vi "resonant.display queue to fp display_MD.vi"() -> ()   [LabVIEW 2012]
uses:
  <vilib>/Utility/VariantDataType/Type.ctl
  GFG/GFGnumericGet.vi
  GFG/GFGbooleanGet.vi
  GFG/GFGImageRefsGet.vi
  GFG/GFGDisplayRefsGet.vi
  GFG/GFG library.lvlib
  <vilib>/Utility/VariantDataType/VariantType.lvlib
panel:
  out "error out 3":errorcluster
  out "error out 2":errorcluster
  out "size(s)":i32[](array[numeric])
  out "# elements in display data queue":i32
  out "error out":errorcluster
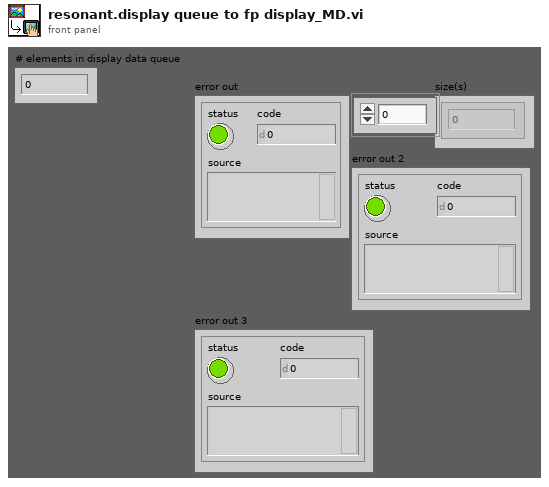
[diagram p1: front panel]
types:
  T1 = cluster{"NewVal":bool, "Event Registration Refnum":refnum<event-registration>}
  T2 = cluster{"Channel 1 small":refnum<vi>, "Channel 2 small":refnum<vi>, "Channel 3 small":refnum<vi>, "Channel 4 small":refnum<vi>, "Channel 1 large":refnum<vi>, "Channel 2 large":refnum<vi>, "Channel 3 large":refnum<vi>, "Channel 4 large":refnum<vi>, "RGB overlay":refnum<vi>, "ROI Image display":refnum<vi>, "arb line scan display":refnum<vi>, "Channel 5 large":refnum<vi>}
  T3 = typedef "IMAQ Image.ctl" = refnum<image>
  T4 = cluster{"Channel 1 small":T3, "Channel 2 small":T3, "Channel 3 small":T3, "Channel 4 small":T3, "Channel 1 large":T3, "Channel 2 large":T3, "Channel 3 large":T3, "Channel 4 large":T3, "RGB overlay":T3, "ROI Image display":T3, "arb line scan display":T3, "Channel 5 large":T3}
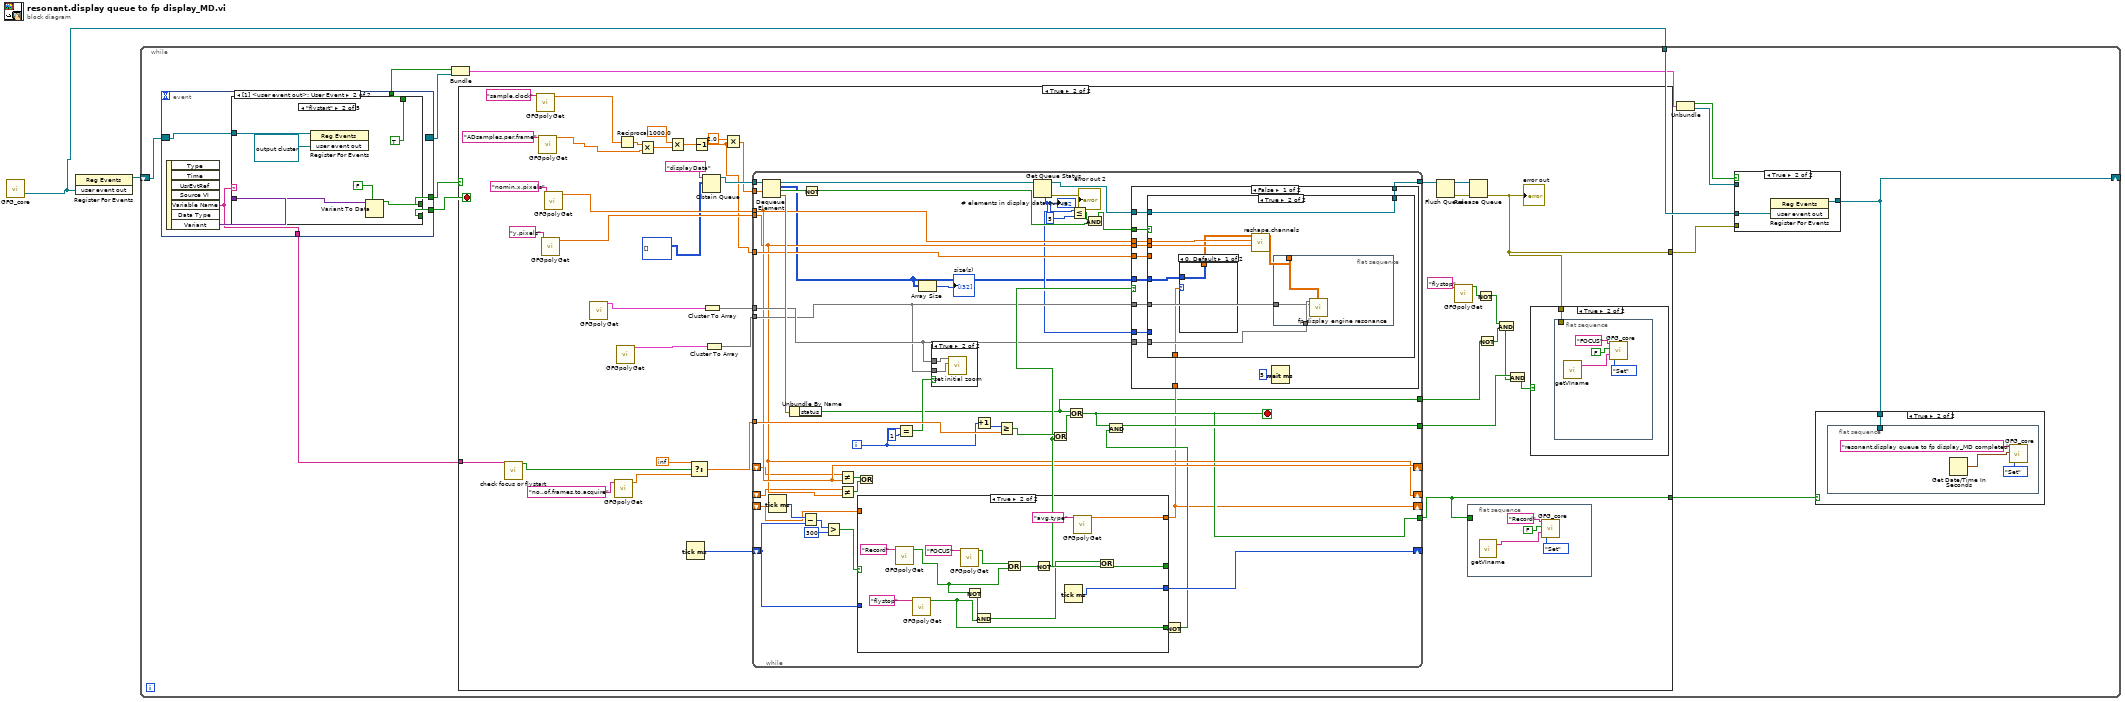
[diagram p0: block diagram]
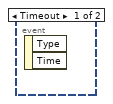
[diagram p4: hidden frame]
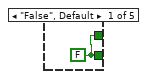
[diagram p5: hidden frame]
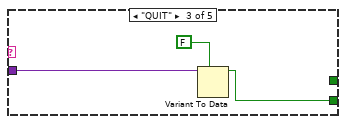
[diagram p6: hidden frame]
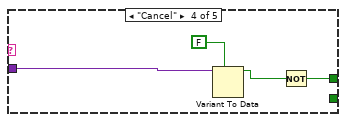
[diagram p7: hidden frame]
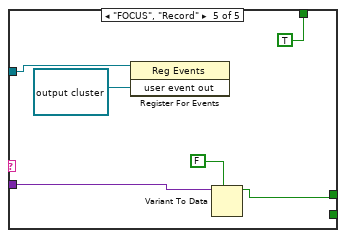
[diagram p8: hidden frame]
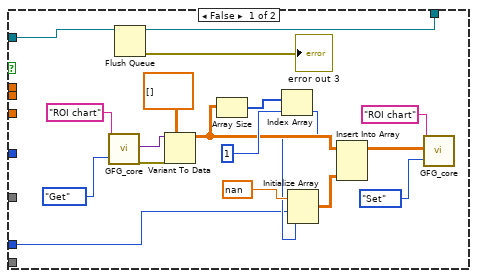
[diagram p12: hidden frame]
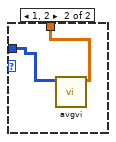
[diagram p13: hidden frame]
diagram:
  n1 = call "GFG_core.vi"() -> ("user event out"=w2:refnum<user-event>)  [unwired: 13 in, 6 out]
  n2 = register-events(w2) -> (reference out=w1:refnum<event-registration>)  [unwired: 2 in, 1 out]
  n3 = while {
    shift-right: [w3] -> _
    shift-left: w1 -> [w11]
    tunnel: w2 -> [w13]
    stop <- w14 stop-if-true
    n4 = event shown="[1] <user event out>: User Event" {
      selector: w11 -> [_ w24]
      dyn-events: [_ _] -> w9
      timeout: _ -> [_ _]
      tunnel: [_ w28] -> w15
      tunnel: [_ w27] -> w14
      tunnel: [_ w25] -> w5
      tunnel: [_ w23] -> w10
      event Timeout {
        n5 = event-data() -> ()  [unwired: 1 in, 2 out]
      }
      event User Event {
        n6 = event-data() -> ("Variable Name"=w25:string, "Variant"=w26:variant)  [unwired: 1 in, 5 out]
        n7 = case shown="\"flystart\"" w25 {
          tunnel: [w29 w33 _ w39 w46] -> w28
          tunnel: [w29 _ w36 _ _] -> w27
          tunnel: w26 -> [_ w34 w38 w41 w47]
          tunnel: w24 -> [_ w31 _ _ w44]
          tunnel: [_ TRUE ("NewVal") _ _ TRUE ("NewVal")] -> w23
          frame "False", Default {
            w29 = FALSE ("NewVal")
          }
          frame "flystart" {
            n8 = register-events(reference=w31, refnum<user-event> refnum ("user event out")) -> ()  [unwired: 1 in, 2 out]
            n9 = Variant To Data(type=FALSE ("NewVal"), Variant=w34) -> (data=w33:bool)  [unwired: 1 in, 1 out]
          }
          frame "QUIT" {
            n10 = Variant To Data(type=FALSE ("NewVal"), Variant=w38) -> (data=w36:bool)  [unwired: 1 in, 1 out]
          }
          frame "Cancel" {
            n11 = Variant To Data(type=FALSE ("NewVal"), Variant=w41) -> (data=w40:bool)  [unwired: 1 in, 1 out]
            n12 = Not(x=w40) -> (.not. x?=w39:bool)
          }
          frame "FOCUS", "Record" {
            n13 = register-events(reference=w44, refnum<user-event> refnum ("user event out")) -> ()  [unwired: 1 in, 2 out]
            n14 = Variant To Data(type=FALSE ("NewVal"), Variant=w47) -> (data=w46:bool)  [unwired: 1 in, 1 out]
          }
        }
      }
    }
    n15 = Bundle("NewVal"=w10, "Event Registration Refnum"=w9) -> (w8:T1)  [unwired: 1 in]
    n16 = case shown="True" w15 {
      tunnel: [_ w59] -> w12
      tunnel: w5 -> [_ w61]
      tunnel: [_ w49] -> w4
      frame False {
      }
      frame True {
        n17 = call "check focus or flystart.vi"("x"=w61) -> ("x .or. y?"=w60:bool)  [unwired: 10 in]
        n18 = call-poly "GFGpolyGet.vi"("Variable Name in"="sample.clock" ("Tag in")) -> ("Numeric"=w82:dbl)  [unwired: 9 in, 1 out]
        n19 = call-poly "GFGpolyGet.vi"("Variable Name in"="ADsamples.per.frame" ("Tag in")) -> ("Numeric"=w67:dbl)  [unwired: 9 in, 1 out]
        n20 = call-poly "GFGpolyGet.vi"("Variable Name in"="y.pixels") -> ("Numeric"=w69:dbl)  [unwired: 9 in, 1 out]
        n21 = call-poly "GFGpolyGet.vi"("Variable Name in"="nomin.x.pixels") -> ("Numeric"=w70:dbl)  [unwired: 9 in, 1 out]
        n22 = call-poly "GFGpolyGet.vi"() -> ("DisplayRefsOut(generic class)"=w79:T2)  [unwired: 10 in, 1 out]
        n23 = call-poly "GFGpolyGet.vi"("Variable Name in"="no..of.frames.to.acquire" ("Tag in")) -> ("Numeric"=w63:dbl)  [unwired: 9 in, 1 out]
        n24 = call-poly "GFGpolyGet.vi"() -> ("Image Refs Out"=w78:T4)  [unwired: 10 in, 1 out]
        n25 = Reciprocal(x=w82) -> (1/x=w87:dbl)
        n26 = Multiply(x=w87, y=w67) -> (x*y=w86:dbl)
        n27 = Multiply(x=1000.0, y=w86) -> (x*y=w84:dbl)
        n28 = Tick Count (ms)() -> (millisecond timer value=w68:u32)
        n29 = Select(t=inf, s=w60, f=w63) -> (s? t:f=w62:dbl)
        n30 = Decrement(x=w84) -> (x-1=w66:dbl)
        n31 = Obtain Queue(name (unnamed)="displayData", element data type=i16[][] [] ("initialized array")) -> (queue out=w80:refnum<queue>)  [unwired: 3 in, 2 out]
        n32 = Cluster To Array(cluster=w79) -> (array=w76:refnum<vi>[])
        n33 = Cluster To Array(cluster=w78) -> (array=w77:T3[])
        n34 = Multiply(x=2.0, y=w66) -> (x*y=w75:dbl)
        n35 = while {
          tunnel: [w110] -> w73
          tunnel: w62 -> [w144]
          tunnel: w75 -> [w140]
          tunnel: w80 -> [w141]
          tunnel: w76 -> [w127]
          tunnel: w77 -> [w119]
          tunnel: w70 -> [w115]
          tunnel: w69 -> [w114]
          shift-right: [w133] -> _
          shift-left: w68 -> [w132]
          tunnel: w66 -> [w126]
          shift-right: [w115] -> _
          shift-left: _ -> [w113]
          shift-right: [w114] -> _
          shift-left: _ -> [w112]
          tunnel: [w104] -> w49
          tunnel: [w107] -> w58
          shift-right: [w103] -> _
          shift-left: _ -> [w102]
          tunnel: [w101] -> w51
          i -> [w130]
          stop <- w104 stop-if-true
          n36 = Dequeue Element(queue=w141, timeout in ms (-1)=w140) -> (queue out=w139:refnum<queue>, element=w100:i16[][], timed out?=w121:bool, error out=w143:errorcluster)  [unwired: 1 in]
          n37 = Tick Count (ms)() -> (millisecond timer value=w137:u32)
          n38 = Unbundle By Name(w143) -> ("status"=w101:bool)
          n39 = Subtract(x=w137, y=w132) -> (x-y=w136:u32)
          n40 = Not(x=w121) -> (.not. x?=w120:bool)
          n41 = Greater?(x=w136, y=u32 300) -> (0:w134:bool)
          n42 = Not Equal?(x=w113, y=w115) -> (x != y?=w117:bool)
          n43 = Not Equal?(x=w112, y=w114) -> (x != y?=w116:bool)
          n44 = case shown="True" w134 {
            tunnel: [_ w199] -> w131
            tunnel: [w194 w203] -> w133
            tunnel: w132 -> [w194 _]
            tunnel: [_ w195] -> w106
            tunnel: [w193 w196] -> w103
            tunnel: w102 -> [w193 _]
            frame False {
            }
            frame True {
              n45 = call-poly "GFGpolyGet.vi"("Variable Name in"="Record") -> ("Boolean"=w200:bool)  [unwired: 10 in]
              n46 = call-poly "GFGpolyGet.vi"("Variable Name in"="flystop") -> ("Boolean"=w195:bool)  [unwired: 10 in]
              n47 = call-poly "GFGpolyGet.vi"("Variable Name in"="FOCUS") -> ("Boolean"=w207:bool)  [unwired: 10 in]
              n48 = Not(x=w200) -> (.not. x?=w201:bool)
              n49 = And(x=w201, y=w195) -> (x .and. y?=w198:bool)
              n50 = Or(x=w207, y=w200) -> (x .or. y?=w208:bool)
              n51 = Not(x=w208) -> (.not. x?=w204:bool)
              n52 = Tick Count (ms)() -> (millisecond timer value=w203:u32)
              n53 = call-poly "GFGpolyGet.vi"("Variable Name in"="avg.type") -> ("Numeric"=w196:dbl)  [unwired: 9 in, 1 out]
              n54 = Or(x=w198, y=w204) -> (x .or. y?=w199:bool)
            }
          }
          n55 = Or(x=w117, y=w116) -> ()  [unwired: 1 out]
          n56 = Equal?(x=w130, y=1) -> (x = y?=w128:bool)
          n57 = Array Size(array=w100) -> (size(s)=→"size(s)":i32[])
          n58 = case shown="True" w128 {
            tunnel: w127 -> [_ w146]
            tunnel: w119 -> [_ w145]
            frame False {
            }
            frame True {
              n59 = call "set initial zoom.vi"("Image Refs In"=w145, "DisplayRefsIn(generic class)"=w146) -> ()  [unwired: 10 in]
            }
          }
          n60 = Increment(x=w130) -> (x+1=w138:i32)
          n61 = Greater Or Equal?(x=w138, y=w144) -> (x >= y?=w142:bool)
          n62 = Get Queue Status(queue=w139) -> (queue out=w111:refnum<queue>, error out=→"error out 2":errorcluster, # elements in queue=w109:i32)  [unwired: 2 in, 5 out]
          "# elements in display data queue" <- w109
          n63 = Or(x=w142, y=w131) -> (x .or. y?=w108:bool)
          n64 = Or(x=w101, y=w108) -> (x .or. y?=w104:bool)
          n65 = Less Or Equal?(x=w109, y=5) -> (x <= y?=w124:bool)
          n66 = And(x=w124, y=w120) -> (x .and. y?=w122:bool)
          n67 = case shown="False" w131 {
            tunnel: w115 -> [w158 _]
            tunnel: w114 -> [w157 _]
            tunnel: w100 -> [w156 _]
            tunnel: w127 -> [w155 _]
            tunnel: w119 -> [w154 _]
            tunnel: w126 -> [w153 _]
            tunnel: w122 -> [w152 _]
            tunnel: w111 -> [w151 w192]
            tunnel: [w150 w192] -> w110
            tunnel: w109 -> [w149 _]
            tunnel: w103 -> [w147 _]
            frame False {
              n68 = case shown="True" w152 {
                tunnel: w158 -> [_ w185]
                tunnel: w157 -> [_ w184]
                tunnel: w156 -> [_ w183]
                tunnel: w155 -> [_ w181]
                tunnel: w154 -> [_ w180]
                tunnel: w153 -> [_ _]
                tunnel: w151 -> [w163 w179]
                tunnel: [w161 w179] -> w150
                tunnel: w149 -> [w159 _]
                tunnel: w147 -> [_ w178]
                frame False {
                  n69 = call "GFG_core.vi"("Variable Name in"="ROI chart", "Action"=enum16{"Init", "Set", "Get"}."Get") -> ("Variant Out"=w173:variant, "error out"=w174:errorcluster)  [unwired: 11 in, 5 out]
                  n70 = Flush Queue(queue=w163) -> (queue out=w161:refnum<queue>, error out=→"error out 3":errorcluster)  [unwired: 1 in, 1 out]
                  n71 = Variant To Data(error in=w174, type=sgl[][] [] ("y backward image"), Variant=w173) -> (data=w169:sgl[][])  [unwired: 1 out]
                  n72 = Array Size(array=w169) -> (size(s)=w167:i32[])
                  n73 = Index Array(array=w167, index=1) -> (element=w160:i32)
                  n74 = Initialize Array(nan, w159, w160) -> (w168:dbl[][])
                  n75 = Insert Into Array(array=w169, new element=w168) -> (w164:sgl[][])  [unwired: 2 in]
                  n76 = call "GFG_core.vi"("Variable Name in"="ROI chart", "Variant in"=w164, "Action"=enum16{"Init", "Set", "Get"}."Set") -> ()  [unwired: 10 in, 7 out]
                }
                frame True {
                  n77 = case shown="0, Default" w178 {
                    tunnel: w183 -> [w189 w191]
                    tunnel: [w189 w190] -> w182
                    frame 0, Default {
                    }
                    frame 1, 2 {
                      n78 = call "avgvi.vi"("image in"=w191) -> ("image out"=w190:sgl[][])  [unwired: 10 in]
                    }
                  }
                  n79 = call "reshape.channels.vi"("y.pixels"=w184, "x.pixels"=w185, "element"=w182) -> ("Array"=w177:dbl[][][])  [unwired: 8 in]
                  n80 = flat-sequence {
                    tunnel: w177 -> [w188]
                    tunnel: w181 -> [w187]
                    tunnel: w180 -> [w186]
                    frame #0 {
                      n81 = call "fp display engine resonance.vi"("channel data in"=w188, "Image Refs In"=w186, "DisplayRefsIn(generic class)"=w187) -> ()  [unwired: 9 in]
                    }
                  }
                }
              }
              n82 = Wait (ms)(milliseconds to wait=u32 5) -> ()  [unwired: 1 out]
            }
            frame True {
            }
          }
          n83 = Not(x=w106) -> (.not. x?=w105:bool)
          n84 = And(x=w104, y=w105) -> (x .and. y?=w107:bool)
        }
        n85 = Flush Queue(queue=w73) -> (queue out=w90:refnum<queue>, error out=w89:errorcluster)  [unwired: 1 in, 1 out]
        n86 = call-poly "GFGpolyGet.vi"("Variable Name in"="flystop") -> ("Boolean"=w53:bool)  [unwired: 10 in]
        n87 = flat-sequence {
          tunnel: w49 -> [_]
          frame #0 {
            n88 = call "getVIname.vi"() -> ("VI name"=w91:string)  [unwired: 19 in]
            n89 = call "GFG_core.vi"("Variable Name in"="Record" ("Tag in"), "Variant in"=FALSE, "Source VI"=w91, "Action"=enum16{"Init", "Set", "Get"}."Set") -> ()  [unwired: 9 in, 7 out]
          }
        }
        n90 = Release Queue(queue=w90, error in (no error)=w89) -> (error out=w59:errorcluster)  [unwired: 1 in, 2 out]
        "error out" <- w59
        n91 = Not(x=w53) -> (.not. x?=w55:bool)
        n92 = Not(x=w51) -> (.not. x?=w50:bool)
        n93 = And(x=w55, y=w50) -> (x .and. y?=w52:bool)
        n94 = And(x=w58, y=w52) -> (x .and. y?=w56:bool)
        n95 = case shown="True" w56 {
          tunnel: w59 -> [_ w95]
          frame False {
          }
          frame True {
            n96 = flat-sequence {
              tunnel: w95 -> [_]
              frame #0 {
                n97 = call "getVIname.vi"() -> ("VI name"=w96:string)  [unwired: 19 in]
                n98 = call "GFG_core.vi"("Variable Name in"="FOCUS" ("Tag in"), "Variant in"=FALSE, "Source VI"=w96, "Action"=enum16{"Init", "Set", "Get"}."Set") -> ()  [unwired: 9 in, 7 out]
              }
            }
          }
        }
      }
    }
    n99 = Unbundle(w8) -> ("NewVal"=w7:bool, "Event Registration Refnum"=w6:refnum<event-registration>)
    n100 = case shown="True" w7 {
      tunnel: [w20 w22] -> w3
      tunnel: w13 -> [_ w21]
      tunnel: w12 -> [_ _]
      tunnel: w6 -> [w20 _]
      frame False {
      }
      frame True {
        n101 = register-events(w21) -> (reference out=w22:refnum<event-registration>)  [unwired: 2 in, 1 out]
      }
    }
    n102 = case shown="True" w4 {
      tunnel: w3 -> [_ w16]
      frame False {
      }
      frame True {
        n103 = flat-sequence {
          tunnel: w16 -> [_]
          frame #0 {
            n104 = Get Date/Time In Seconds() -> (seconds since 1Jan1904=w17:timestamp)
            n105 = call "GFG_core.vi"("Variable Name in"="resonant.display queue to fp display_MD completed", "Variant in"=w17, "Action"=enum16{"Init", "Set", "Get"}."Set") -> ()  [unwired: 10 in, 7 out]
          }
        }
      }
    }
  }
